vi "testBench-HookValidationA1.vi"() -> ()   [LabVIEW 2015]
panel:
  in  "quit":bool
  out "quitting":bool
  out "关系图":cluster{i32[], dbl[]}(graph)
  in  "钩子起始角度":dbl=60.0 format="%#_13g"
  in  "槽数":i32=3
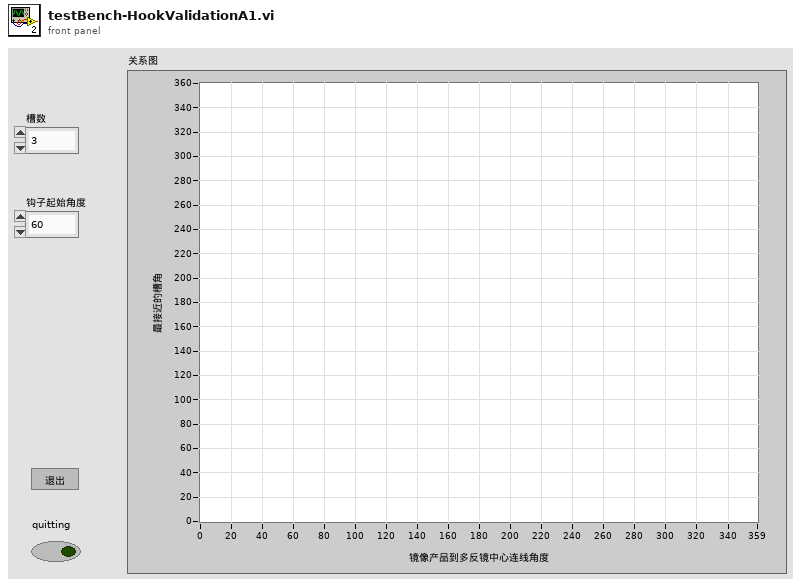
[diagram p1: front panel]
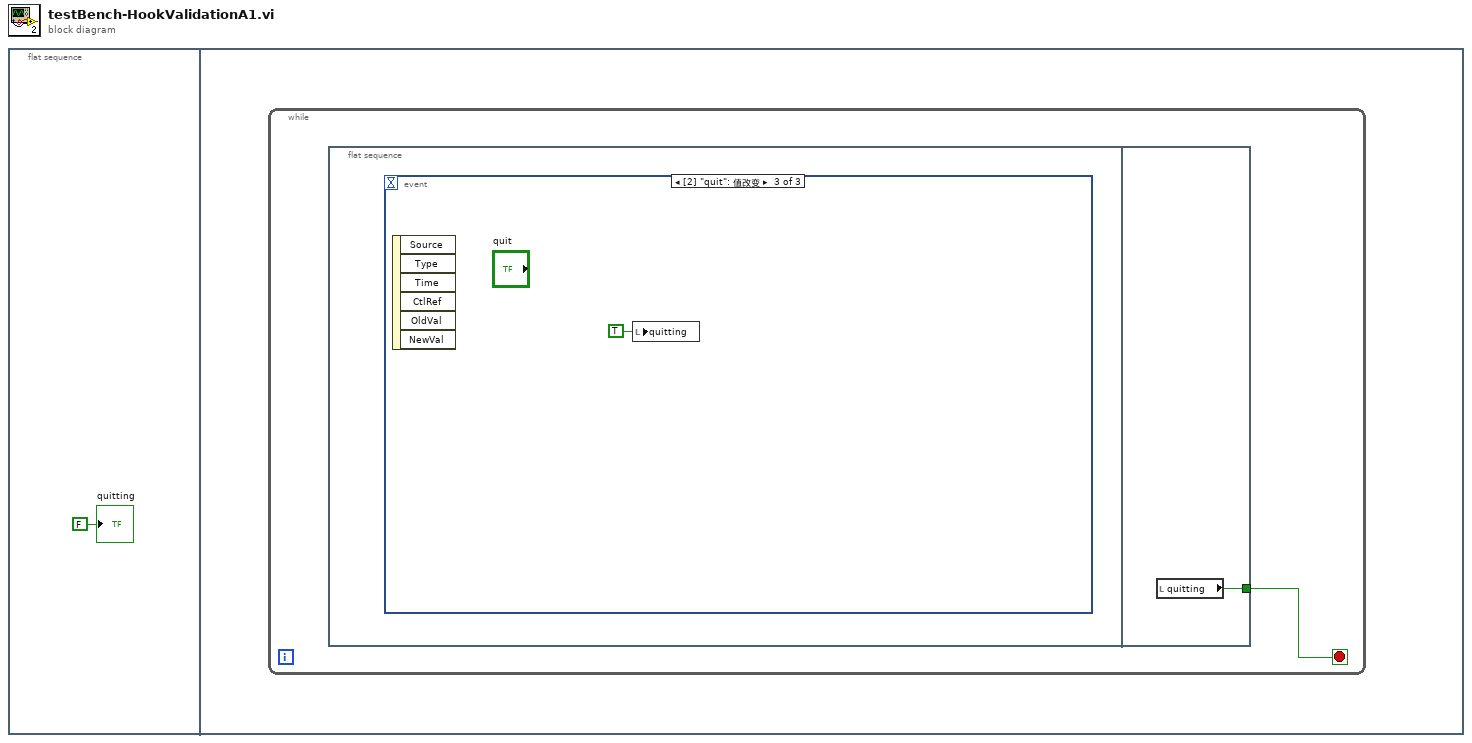
[diagram p0: block diagram]
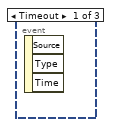
[diagram p2: hidden frame]
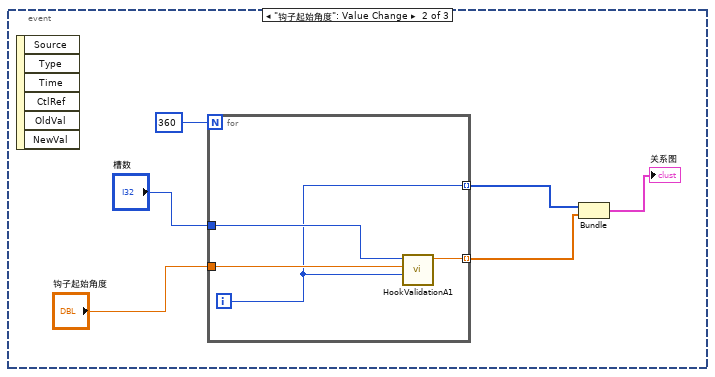
[diagram p3: hidden frame]
diagram:
  n1 = flat-sequence {
    frame #0 {
      "quitting" <- FALSE ("quitting")
    }
    frame #1 {
      n2 = while {
        stop <- w2 stop-if-true
        n3 = flat-sequence {
          tunnel: [w14] -> w2
          frame #0 {
            n4 = event shown="[2] \"quit\": 值改变" {
              selector: _ -> [_ _ _]
              dyn-events: _ -> [_ _ _]
              timeout: _ -> [_ _ _]
              event Timeout {
                n5 = event-data() -> ()  [unwired: 1 in, 3 out]
              }
              event "钩子起始角度": Value Change {
                n6 = event-data() -> ()  [unwired: 1 in, 6 out]
                n7 = for {
                  N: 360 -> [_]
                  tunnel: "槽数" -> [w12]
                  tunnel: "钩子起始角度" -> [w11]
                  tunnel: [w10] -> w7 mode=indexing
                  tunnel: [w9] -> w8 mode=indexing
                  i -> [w9]
                  n8 = call "HookValidationA1.vi"("镜像产品到中心连线角度"=w9, "钩子起始角度"=w11, "槽数"=w12) -> ("最接近槽角"=w10:dbl)  [unwired: 8 in]
                }
                n9 = Bundle(w8, w7) -> (→"关系图":cluster{i32[], dbl[]})  [unwired: 1 in]
              }
              event "quit": Value Change {
                n10 = event-data() -> ()  [unwired: 1 in, 6 out]
                n11 = local write "quitting"(TRUE ("quitting")) -> ()
              }
            }
          }
          frame #1 {
            n12 = local read "quitting"() -> (w14:bool)
          }
        }
      }
    }
  }
